vi "Populate from String.vi"(8 "error in (no error)":errorcluster, 10 "Line in":string, 11 "FlexWorktable in":refnum<class "FlexWorktable.lvclass">) -> (0 "error out":errorcluster, 3 "FlexWorktable out":refnum<class "FlexWorktable.lvclass">)   [LabVIEW 2023, in "FlexWorktable.lvclass"]
uses:
  FlexWorktable.lvclass
  FlexWorktable.lvclass/FlexWorktable.ctl
  <vilib>/Utility/error.llb/Trim Whitespace One-Sided.vi
  <vilib>/regexp/Match Regular Expression.xnode
  Vec3d Class/Vec3d.lvclass
  Orient3d Class/Orient3d.lvclass
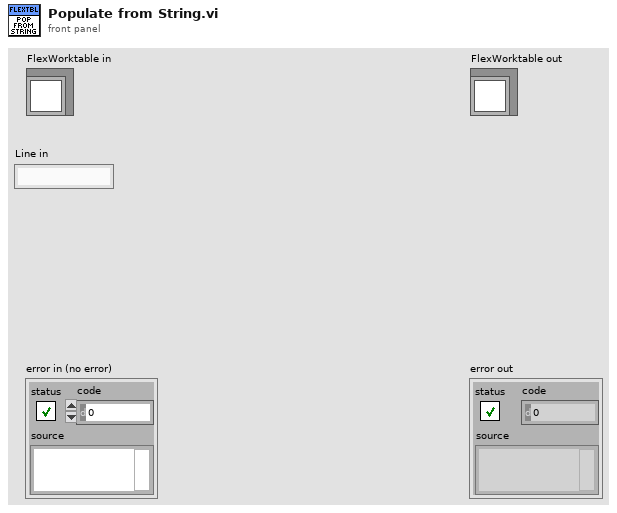
[diagram p1: front panel]
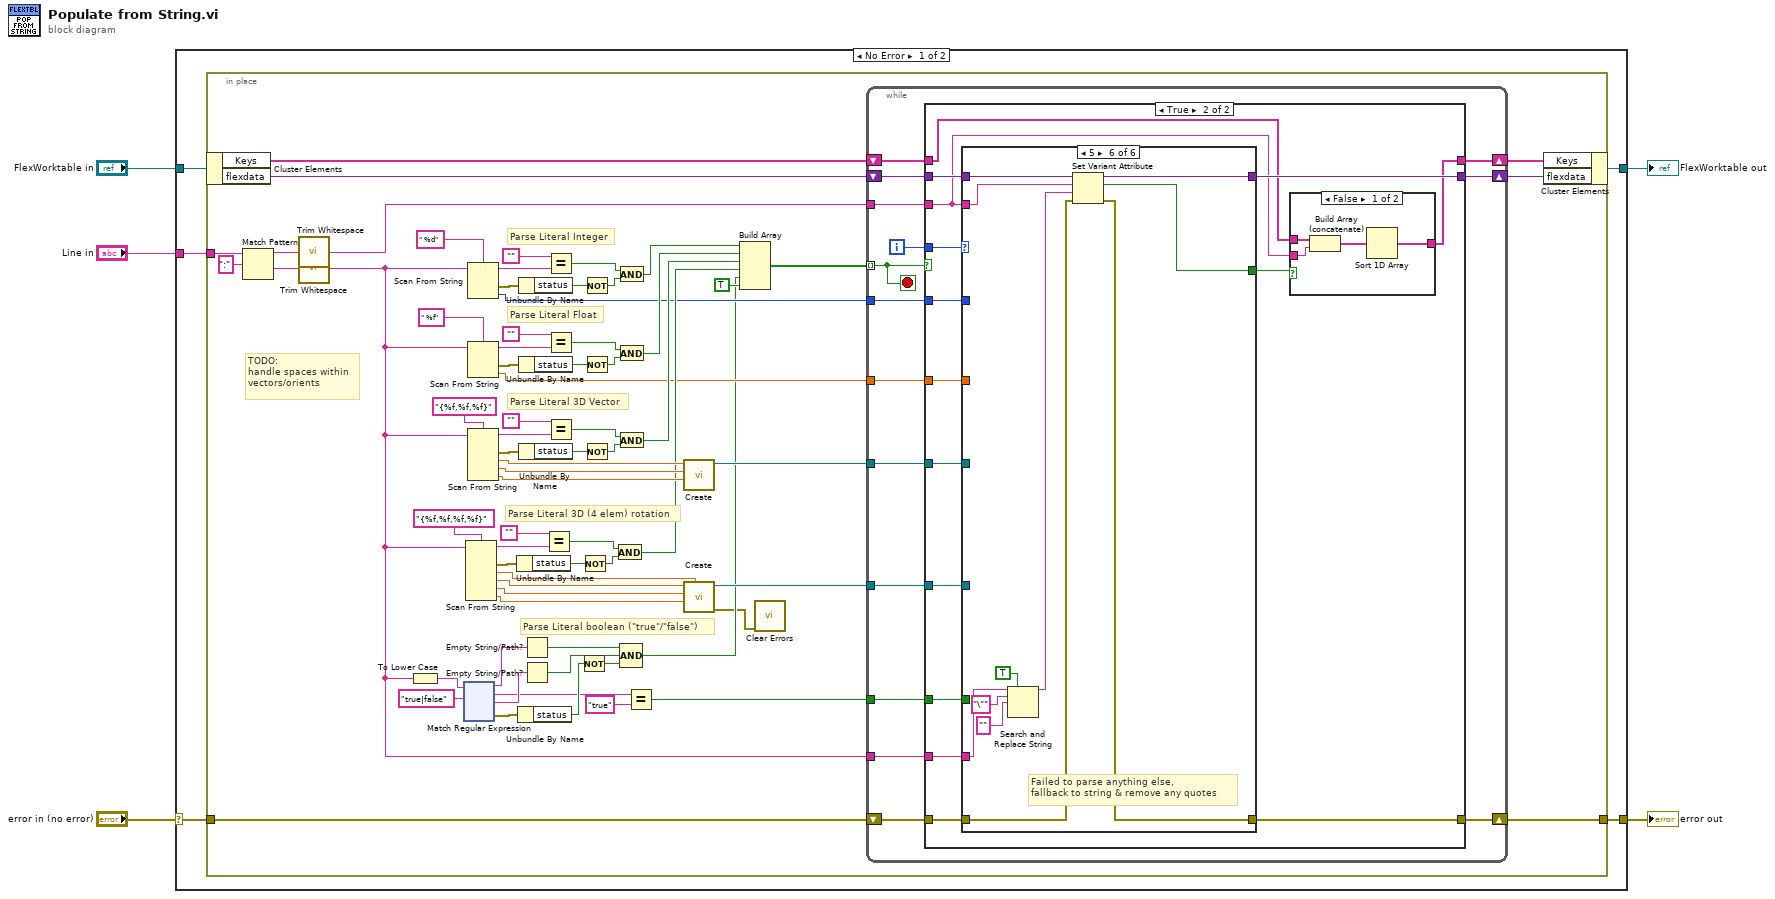
[diagram p0: block diagram]
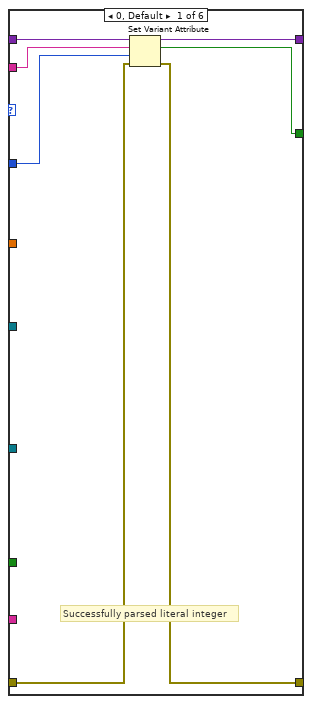
[diagram p4: hidden frame]
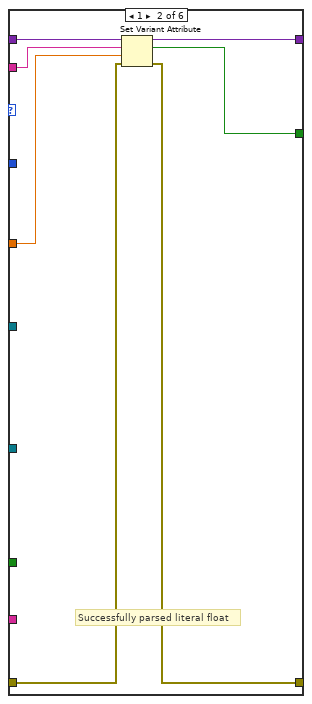
[diagram p5: hidden frame]
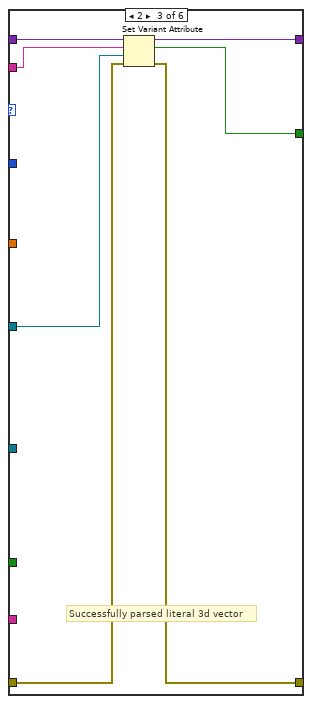
[diagram p6: hidden frame]
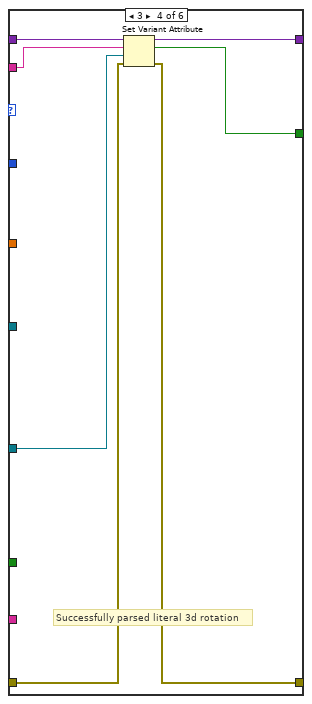
[diagram p7: hidden frame]
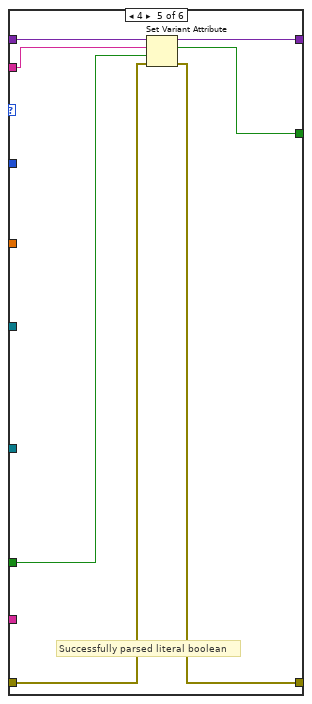
[diagram p8: hidden frame]
diagram:
  n1 = case shown="No Error" "error in (no error)" {
    selector: "error in (no error)" -> [w8 w284]
    tunnel: [w6 w284] -> w4
    tunnel: [w7 w283] -> w2
    tunnel: "FlexWorktable in" -> [w10 w283]
    tunnel: "Line in" -> [w9 _]
    frame No Error {
      n2 = in-place {
        in-place-border: w9 -> [w81]
        in-place-border: w8 -> [w30]
        in-place-border: [w29] -> w6
        # "TODO:\nhandle spaces within\nvectors/orients"
        # "Parse Literal boolean (\"true\"/\"false\")"
        # "Parse Literal 3D (4 elem) rotation"
        # "Parse Literal 3D Vector"
        # "Parse Literal Float"
        # "Parse Literal Integer"
        n3 = in-place-cluster #1(w10) -> ("Keys"=w28:string[], "flexdata"=w33:variant)
        n4 = Match Pattern(string=w81, regular expression=":") -> (before substring=w79:string, after substring=w78:string)  [unwired: 1 in, 2 out]
        n5 = call <vilib>:"Trim Whitespace.vi"("string"=w79) -> ("trimmed string"=w31:string)  [unwired: 1 in]
        n6 = call <vilib>:"Trim Whitespace.vi"("string"=w78) -> ("trimmed string"=w13:string)  [unwired: 1 in]
        n7 = To Lower Case(string=w13) -> (all lower case string=w18:string)
        n8 = xnode "Match Regular Expression"("input string"=w18, "regular expression"="true|false") -> ("before match"=w24:string, "whole match"=w17:string, "after match"=w23:string, "error out"=w25:errorcluster)  [unwired: 4 in, 1 out]
        n9 = Scan From String(format string="{%f,%f,%f,%f}", input string=w13) -> (remaining string=w63:string, error out=w64:errorcluster, output 1=w74:dbl, output 2=w75:dbl, output 3=w76:dbl, output 4=w77:dbl)  [unwired: 6 in, 1 out]
        n10 = Scan From String(format string=" %d", input string=w13) -> (remaining string=w47:string, error out=w48:errorcluster, output 1=w34:i32)  [unwired: 3 in, 1 out]
        n11 = Scan From String(format string=" %f", input string=w13) -> (remaining string=w52:string, error out=w53:errorcluster, output 1=w35:dbl)  [unwired: 3 in, 1 out]
        n12 = Scan From String(format string="{%f,%f,%f}", input string=w13) -> (remaining string=w57:string, error out=w58:errorcluster, output 1=w71:dbl, output 2=w72:dbl, output 3=w73:dbl)  [unwired: 5 in, 1 out]
        n13 = Unbundle By Name(w64) -> ("status"=w66:bool)
        n14 = Unbundle By Name(w25) -> ("status"=w21:bool)
        n15 = Unbundle By Name(w48) -> ("status"=w50:bool)
        n16 = Unbundle By Name(w53) -> ("status"=w55:bool)
        n17 = Unbundle By Name(w58) -> ("status"=w60:bool)
        n18 = Empty String/Path?(string/path=w24) -> (empty?=w22:bool)
        n19 = Empty String/Path?(string/path=w23) -> (empty?=w20:bool)
        n20 = Equal?(x="", y=w63) -> (x = y?=w65:bool)
        n21 = Equal?(x="", y=w47) -> (x = y?=w49:bool)
        n22 = Equal?(x="", y=w52) -> (x = y?=w54:bool)
        n23 = Equal?(x="", y=w57) -> (x = y?=w59:bool)
        n24 = Not(x=w21) -> (.not. x?=w19:bool)
        n25 = Not(x=w66) -> (.not. x?=w67:bool)
        n26 = Not(x=w50) -> (.not. x?=w51:bool)
        n27 = Not(x=w55) -> (.not. x?=w56:bool)
        n28 = Not(x=w60) -> (.not. x?=w61:bool)
        n29 = And(x=w65, y=w67) -> (x .and. y?=w68:bool)
        n30 = And(x=w49, y=w51) -> (x .and. y?=w69:bool)
        n31 = And(x=w54, y=w56) -> (x .and. y?=w70:bool)
        n32 = And(x=w59, y=w61) -> (x .and. y?=w62:bool)
        n33 = Compound Arithmetic op=AND(w22, w20, w19) -> (w14:bool)
        n34 = Equal?(x=w17, y="true") -> (x = y?=w12:bool)
        n35 = call "Create.vi"("Z"=w73, "Y"=w72, "X"=w71) -> ("Vec3d Class out"=w37:refnum<class "Vec3d.lvclass">)  [unwired: 7 in, 1 out]
        n36 = call "Create.vi"("x"=w74, "w"=w77, "z"=w76, "y"=w75) -> ("error out"=w11:errorcluster, "Orient3d out"=w36:refnum<class "Orient3d.lvclass">)  [unwired: 6 in]
        n37 = Build Array(w69, w70, w62, w68, w14, TRUE ("element")) -> (w38:bool[])
        n38 = call <vilib>:"Clear Errors.vi"("error in (no error)"=w11) -> ()  [unwired: 5 in, 2 out]
        n39 = while {
          tunnel: w38 -> [w204] mode=indexing
          tunnel: w37 -> [w208]
          tunnel: w36 -> [w207]
          tunnel: w35 -> [w209]
          tunnel: w34 -> [w210]
          tunnel: w13 -> [w206]
          shift-right: [w211] -> w32
          shift-left: w33 -> [w212]
          tunnel: w31 -> [w205]
          shift-right: [w202] -> w29
          shift-left: w30 -> [w203]
          shift-right: [w200] -> w27
          shift-left: w28 -> [w201]
          tunnel: w12 -> [w199]
          i -> [w213]
          stop <- w204 stop-if-true
          n40 = case shown="True" w204 {
            tunnel: w213 -> [_ w231]
            tunnel: w212 -> [w216 w225]
            tunnel: [w216 w224] -> w211
            tunnel: w210 -> [_ w230]
            tunnel: w209 -> [_ w229]
            tunnel: w208 -> [_ w228]
            tunnel: w207 -> [_ w227]
            tunnel: w206 -> [_ w226]
            tunnel: w205 -> [_ w219]
            tunnel: w203 -> [w215 w223]
            tunnel: [w215 w222] -> w202
            tunnel: w201 -> [w214 w221]
            tunnel: [w214 w218] -> w200
            tunnel: w199 -> [_ w217]
            frame False {
            }
            frame True {
              n41 = case shown="5" w231 {
                tunnel: w230 -> [w240 _ _ _ _ _]
                tunnel: w229 -> [_ w247 _ _ _ _]
                tunnel: w228 -> [_ _ w253 _ _ _]
                tunnel: w227 -> [_ _ _ w261 _ _]
                tunnel: w226 -> [_ _ _ _ _ w273]
                tunnel: w225 -> [w243 w250 w257 w264 w271 w282]
                tunnel: w219 -> [w241 w248 w252 w262 w269 w280]
                tunnel: [w242 w249 w256 w263 w270 w281] -> w224
                tunnel: w223 -> [w239 w246 w255 w260 w267 w279]
                tunnel: [w238 w245 w254 w259 w266 w278] -> w222
                tunnel: [w237 w244 w251 w258 w265 w277] -> w220
                tunnel: w217 -> [_ _ _ _ w268 _]
                frame 0, Default {
                  # "Successfully parsed literal integer"
                  n42 = Set Variant Attribute(Variant=w243, name=w241, value=w240, error in=w239) -> (Variant out=w242:variant, replaced=w237:bool, error out=w238:errorcluster)
                }
                frame 1 {
                  # "Successfully parsed literal float"
                  n43 = Set Variant Attribute(Variant=w250, name=w248, value=w247, error in=w246) -> (Variant out=w249:variant, replaced=w244:bool, error out=w245:errorcluster)
                }
                frame 2 {
                  # "Successfully parsed literal 3d vector"
                  n44 = Set Variant Attribute(Variant=w257, name=w252, value=w253, error in=w255) -> (Variant out=w256:variant, replaced=w251:bool, error out=w254:errorcluster)
                }
                frame 3 {
                  # "Successfully parsed literal 3d rotation"
                  n45 = Set Variant Attribute(Variant=w264, name=w262, value=w261, error in=w260) -> (Variant out=w263:variant, replaced=w258:bool, error out=w259:errorcluster)
                }
                frame 4 {
                  # "Successfully parsed literal boolean"
                  n46 = Set Variant Attribute(Variant=w271, name=w269, value=w268, error in=w267) -> (Variant out=w270:variant, replaced=w265:bool, error out=w266:errorcluster)
                }
                frame 5 {
                  # "Failed to parse anything else,\nfallback to string & remove any quotes"
                  n47 = Search and Replace String(replace all?=TRUE ("replace all? (F)"), input string=w273, search string="\"", replace string="" ("replace string (\"\")")) -> (result string=w272:string)  [unwired: 4 in, 3 out]
                  n48 = Set Variant Attribute(Variant=w282, name=w280, value=w272, error in=w279) -> (Variant out=w281:variant, replaced=w277:bool, error out=w278:errorcluster)
                }
              }
              n49 = case shown="False" w220 {
                tunnel: w221 -> [w235 w236]
                tunnel: w219 -> [w234 _]
                tunnel: [w232 w236] -> w218
                frame False {
                  n50 = Build Array (concatenate)(w235, w234) -> (w233:string[])
                  n51 = Sort 1D Array(array=w233) -> (sorted array=w232:string[])
                }
                frame True {
                }
              }
            }
          }
        }
        n52 = in-place-cluster #1("Keys"=w27, "flexdata"=w32) -> (w7:refnum<class "FlexWorktable.lvclass">)
      }
    }
    frame Error {
    }
  }
  "error out" <- w4
  "FlexWorktable out" <- w2
